vi "Log Tester.vi"() -> ()   [LabVIEW 2021, in "Error_Manager.lvlib" / "LogRotate.lvclass"]
uses:
  LogRotate.lvclass
  LogData.ctl
  LogRotate.lvclass/LogRotate.ctl
panel:
  out "filePath":path
  in  "Data":T1 {"Time Stamp" format="%<%x %.3X>T"}
  in  "Send Data":bool
  in  "size(KB)":u32
  in  "Name":string
  in  "Init":bool
  in  "stop":bool
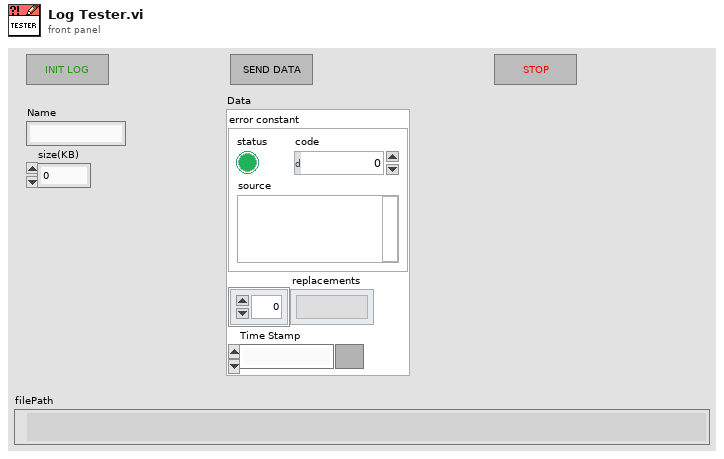
[diagram p1: front panel]
types:
  T1 = typedef "Error_Manager.lvlib/LogRotate.lvclass/LogData.ctl" = cluster{"error constant":errorcluster, "replacements":string[], "Time Stamp":timestamp}
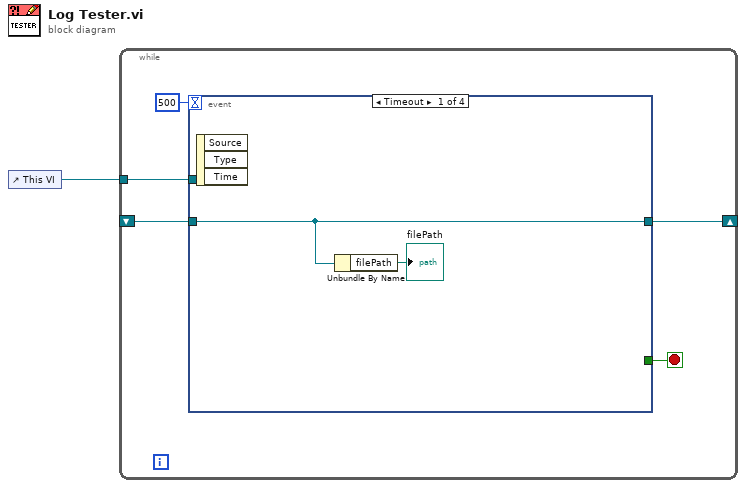
[diagram p0: block diagram]
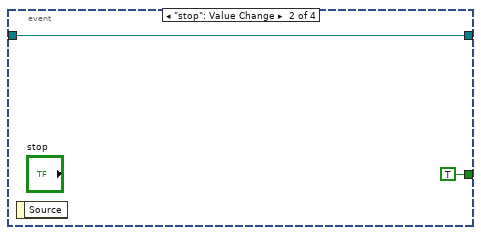
[diagram p2: hidden frame]
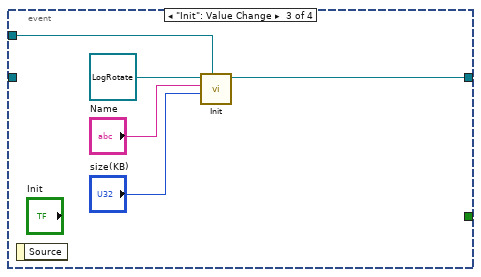
[diagram p3: hidden frame]
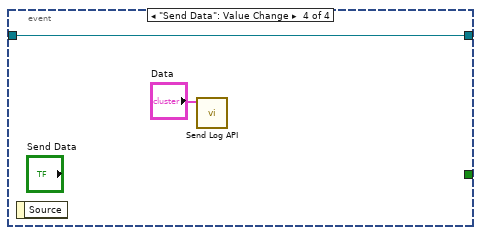
[diagram p4: hidden frame]
diagram:
  n1 = control-ref of="This VI"() -> (w1:refnum<vi>)
  n2 = while {
    tunnel: w1 -> [w4]
    shift-right: [w3] -> _
    shift-left: _ -> [w2]
    stop <- w6 stop-if-true
    n3 = event shown="[0] Timeout" {
      selector: _ -> [_ _ _ _]
      dyn-events: _ -> [_ _ _ _]
      timeout: 500 -> [_ _ _ _]
      tunnel: [_ TRUE ("stop") _ _] -> w6
      tunnel: w4 -> [_ _ w12 _]
      tunnel: [w8 w9 w11 w17] -> w3
      tunnel: w2 -> [w8 w9 _ w17]
      event Timeout {
        n4 = event-data() -> ()  [unwired: 1 in, 3 out]
        n5 = Unbundle By Name(w8) -> ("filePath"=→"filePath":path)
      }
      event "stop": Value Change {
        n6 = event-data() -> ()  [unwired: 1 in, 1 out]
      }
      event "Init": Value Change {
        n7 = event-data() -> ()  [unwired: 1 in, 1 out]
        n8 = call "Init.vi"("TopLevel"=w12, "size(KB)"="size(KB)", "Name"="Name", "LogRotate in"=refnum<class "LogRotate.lvclass"> refnum) -> ("LogRotate out"=w11:refnum<class "LogRotate.lvclass">)  [unwired: 6 in, 1 out]
      }
      event "Send Data": Value Change {
        n9 = event-data() -> ()  [unwired: 1 in, 1 out]
        n10 = call "Send Log API.vi"("Data"="Data") -> ()  [unwired: 10 in, 1 out]
      }
    }
  }
